vi "myPID.vi"(0 "P":dbl=0.9999999999999999 format="%.2f", 1 "I":dbl=1.0 format="%.2f", 2 "D":dbl=0.15 format="%.2f", 3 "set point":dbl=55.0 format="%.2f", 4 "process variable":dbl=22.58241758241758 format="%.2f") -> (5 "output value":dbl=1.0 format="%.2f")   [LabVIEW 2017]
panel:
  in  "low PID param":dbl=10.0
  in  "high PID param.":dbl=10.0
  in  "int upper limit":dbl=0.5
  in  "int lower limit":dbl=-0.05
  out "int":dbl=-2.609670330091651
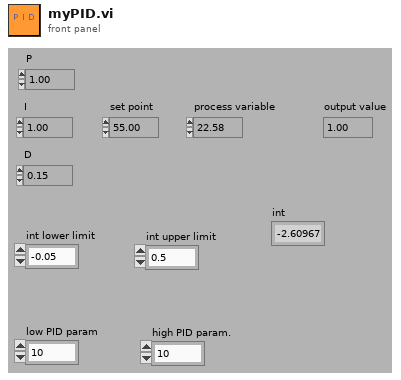
[diagram p1: front panel]
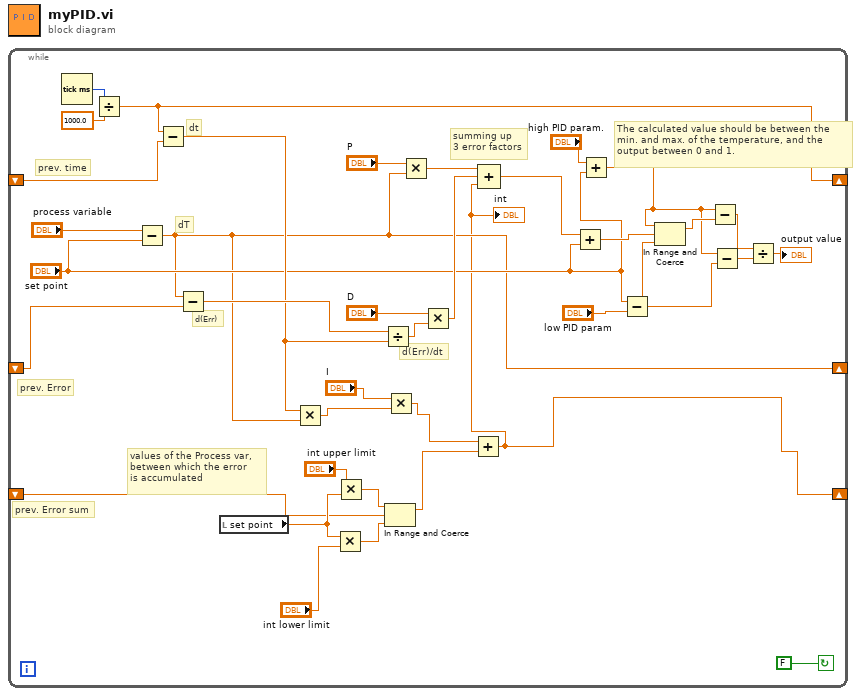
[diagram p0: block diagram]
diagram:
  n1 = while {
    shift-left: _ -> [w33]
    shift-right: [w6] -> _
    shift-left: _ -> [w31]
    shift-right: [w20] -> _
    shift-right: [w5] -> _
    shift-left: _ -> [w15]
    stop <- FALSE continue-if-true
    # "d(Err)/dt"
    # "values of the Process var, \nbetween which the error \nis accumulated"
    # "dT"
    # "The calculated value should be between the \nmin. and max. of the temperature, and the \noutput between 0 and 1."
    # "summing up \n3 error factors"
    # "dt"
    # "prev. Error sum"
    # "d(Err)"
    # "prev. time"
    # "prev. Error"
    n2 = Tick Count (ms)() -> (millisecond timer value=w36:u32)
    n3 = Divide(x=w36, y=1000.0) -> (x/y=w20:dbl)
    n4 = Subtract(x="process variable", y="set point") -> (x-y=w6:dbl)
    n5 = Subtract(x=w20, y=w31) -> (x-y=w19:dbl)
    n6 = Subtract(x=w6, y=w33) -> (x-y=w30:dbl)
    n7 = local read "set point"() -> (w16:dbl)
    n8 = Multiply(x=w19, y=w6) -> (x*y=w14:dbl)
    n9 = Multiply(x=w16, y="int lower limit") -> (x*y=w17:dbl)
    n10 = Multiply(x="int upper limit", y=w16) -> (x*y=w18:dbl)
    n11 = Divide(x=w30, y=w19) -> (x/y=w35:dbl)
    n12 = In Range and Coerce(upper limit=w18, x=w15, lower limit=w17) -> (coerced(x)=w11:dbl)  [unwired: 1 out]
    n13 = Multiply(x="I", y=w14) -> (x*y=w13:dbl)
    n14 = Multiply(x="P", y=w6) -> (x*y=w22:dbl)
    n15 = Multiply(x="D", y=w35) -> (x*y=w32:dbl)
    n16 = Add(x=w13, y=w11) -> (x+y=w5:dbl)
    "int" <- w5
    n17 = Compound Arithmetic op=ADD(w22, w32, w5) -> (w23:dbl)
    n18 = Add(x=w23, y="set point") -> (x+y=w29:dbl)
    n19 = Add(x="high PID param.", y="set point") -> (x+y=w9:dbl)
    n20 = Subtract(x="set point", y="low PID param") -> (x-y=w10:dbl)
    n21 = In Range and Coerce(upper limit=w9, x=w29, lower limit=w10) -> (coerced(x)=w26:dbl)  [unwired: 1 out]
    n22 = Subtract(x=w9, y=w26) -> (x-y=w24:dbl)
    n23 = Subtract(x=w9, y=w10) -> (x-y=w25:dbl)
    n24 = Divide(x=w24, y=w25) -> (x/y=→"output value":dbl)
  }
